vi "set_calibration_image(subVI).vi"(6 "error in (no error)":errorcluster, 9 "File Path":path, 10 "Calibration Axis Info":T2={"Origin Pixel"={"X"=0.0, "Y"=0.0}, "Angle Relative to Horizontal (deg)"=0.0, "Axis Reference"=1} {"Axis Reference" items=["Direct", "Indirect"]; "Angle Relative to Horizontal (deg)" format="%.2f"; "Origin Pixel"."Y" format="%.2f"; "Origin Pixel"."X" format="%.2f"}, 11 "Image Dst":T1) -> (3 "calib image":T1, 4 "error out":errorcluster, 5 "Image Out":T1)   [LabVIEW 2020]
uses:
  <vilib>/vision/Image Controls.llb/IMAQ Image.ctl
  <vilib>/vision/NI_Vision_Development_Module.lvlib
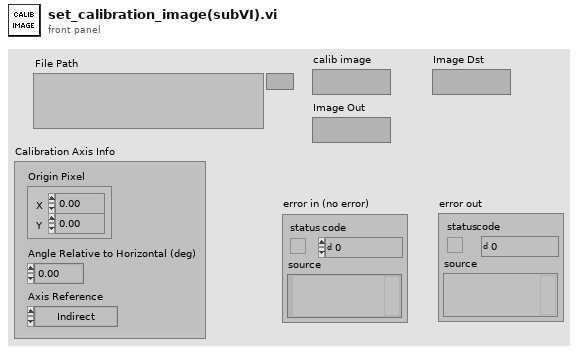
[diagram p1: front panel]
types:
  T1 = typedef "IMAQ Image.ctl" = refnum<image>
  T2 = cluster{"Origin Pixel":cluster{"X":sgl, "Y":sgl}, "Angle Relative to Horizontal (deg)":sgl, "Axis Reference":u32}
  T3 = cluster{"Origin Pixel":cluster{"X":sgl, "Y":sgl}, "Angle Relative to Horizontal (deg)":sgl, "X Axis Pixel":cluster{"X":sgl, "Y":sgl}, "Axis Reference":u32}
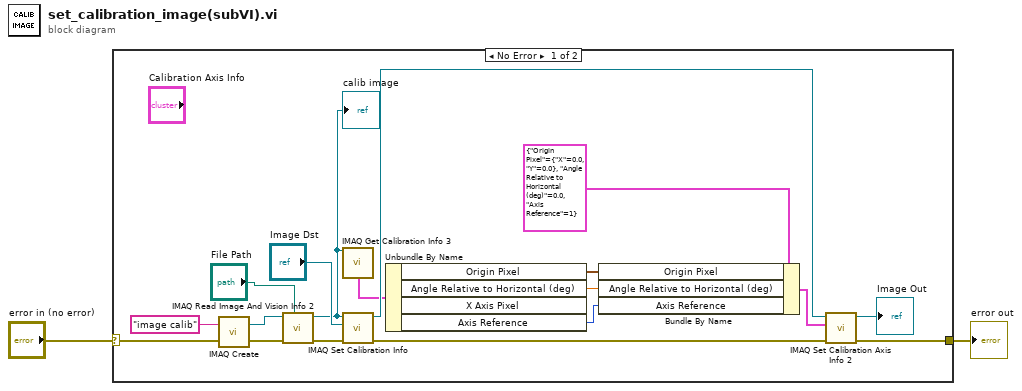
[diagram p0: block diagram]
diagram:
  n1 = case shown="No Error" "error in (no error)" {
    selector: "error in (no error)" -> [w13 w21]
    tunnel: [w11 w21] -> w2
    frame No Error {
      n2 = call "IMAQ Create"("Image Name"="image calib", "error in (no error)"=w13) -> ("New Image"=w15:T1, "error out"=w16:errorcluster)  [unwired: 3 in]
      n3 = call "IMAQ Read Image And Vision Info 2"("File Path"="File Path", "error in (no error)"=w16, "Image"=w15) -> ("error out"=w20:errorcluster, "Image Out"=w9:T1)  [unwired: 6 in, 1 out]
      "calib image" <- w9
      n4 = call "IMAQ Get Calibration Info 3"("Calibration Template Image"=w9) -> ("Calibration Axis Info"=w8:T3)  [unwired: 6 in, 8 out]
      n5 = call "IMAQ Set Calibration Info"("error in (no error)"=w20, "Image Dst"="Image Dst", "Image Src"=w9) -> ("error out"=w17:errorcluster, "Calibrated Image"=w10:T1)  [unwired: 7 in]
      n6 = Unbundle By Name(w8) -> ("Origin Pixel"=w6:cluster{"X":sgl, "Y":sgl}, "Angle Relative to Horizontal (deg)"=w5:sgl, "Axis Reference"=w4:u32)  [unwired: 1 out]
      n7 = Bundle By Name(cluster=T2 {"Origin Pixel"={"X"=0.0, "Y"=0.0}, "Angle Relative to Horizontal (deg)"=0.0, "Axis Reference"=1} ("Calibration Axis Info"), "Origin Pixel"=w6, "Angle Relative to Horizontal (deg)"=w5, "Axis Reference"=w4) -> (w3:T2)
      n8 = call-poly "IMAQ Set Calibration Axis Info 2"("error in (no error)"=w17, "Calibration Axis Info"=w3, "Calibration Template Image In"=w10) -> ("error out"=w11:errorcluster, "Calibration Template Image Out"=→"Image Out":T1)  [unwired: 7 in]
    }
    frame Error {
    }
  }
  "error out" <- w2
